vi "stage_move_axis_absolute.vi"(3 "error in":errorcluster, 4 "Ziel xyz IN [mm]":dbl[](array[numeric]), 5 "Achse":i32) -> (0 "error out":errorcluster, 1 "Fertig?":bool, 2 "Ziel xyz OUT [mm]":dbl[](array[numeric]))   [LabVIEW 2009]
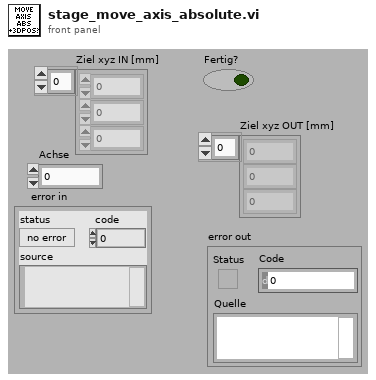
[diagram p1: front panel]
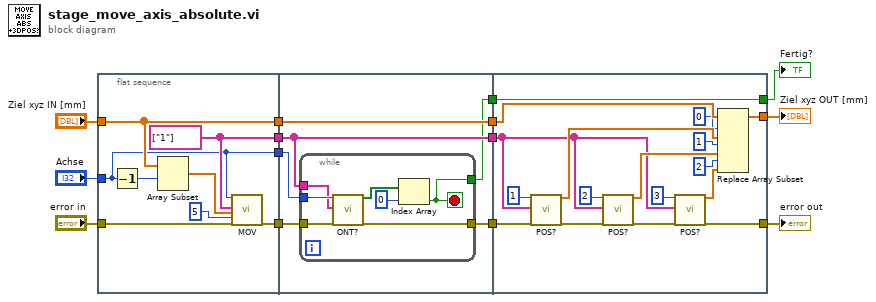
[diagram p0: block diagram]
diagram:
  n1 = flat-sequence {
    tunnel: [w16] -> w14
    tunnel: [w22] -> w13
    tunnel: "Achse" -> [w16]
    tunnel: [w20] -> w12
    tunnel: [w18] -> w7
    tunnel: "Ziel xyz IN [mm]" -> [w18]
    tunnel: "error in" -> [w15]
    tunnel: w14 -> [w28]
    tunnel: w13 -> [w27]
    tunnel: [w26] -> w11
    tunnel: w12 -> [w25]
    tunnel: [w25] -> w10
    tunnel: w7 -> [w24]
    tunnel: [w24] -> w6
    tunnel: [w23] -> w2
    tunnel: w11 -> [w52]
    tunnel: w10 -> [w37]
    tunnel: w6 -> [w49]
    tunnel: [w50] -> w9
    tunnel: [w46] -> w3
    tunnel: w2 -> [w36]
    tunnel: [w36] -> w1
    frame #0 {
      w20 = string[] ["1"] ("Axes to move")
      n2 = Decrement(x=w16) -> (x-1=w17:i32)
      n3 = Array Subset(array=w18, index=w17) -> (w19:dbl[])  [unwired: 1 in]
      n4 = call "MOV.vi"("System no."=w16, "Axes to move"=w20, "Position values"=w19, "No.of digits"=i16 5, "error in"=w15) -> ("error out"=w22:errorcluster)  [unwired: 14 in]
    }
    frame #1 {
      n5 = while {
        tunnel: w28 -> [w35]
        tunnel: w27 -> [w34]
        tunnel: [w33] -> w26
        tunnel: w25 -> [w32]
        tunnel: [w29] -> w23
        stop <- w29 stop-if-true
        n6 = call "ONT?.vi"("System no."=w35, "Axes to query"=w32, "error in"=w34) -> ("Axis on target?"=w30:bool[], "error out"=w33:errorcluster)  [unwired: 15 in]
        n7 = Index Array(array=w30, index=0 ("Index")) -> (element=w29:bool)
      }
    }
    frame #2 {
      n8 = call "POS?.vi"("System no."=1, "Axes to query"=w37, "error in"=w52) -> ("Position"=w51:dbl[], "error out"=w48:errorcluster)  [unwired: 15 in]
      n9 = call "POS?.vi"("System no."=2, "Axes to query"=w37, "error in"=w48) -> ("Position"=w39:dbl[], "error out"=w47:errorcluster)  [unwired: 15 in]
      n10 = call "POS?.vi"("System no."=3, "Axes to query"=w37, "error in"=w47) -> ("Position"=w38:dbl[], "error out"=w46:errorcluster)  [unwired: 15 in]
      n11 = Replace Array Subset(array=w49, new element #1=w51, index #1=0 ("Index"), new element #2=w39, index #2=1 ("Index"), new element #3=w38, index #3=2 ("Index")) -> (w50:dbl[])
    }
  }
  "Ziel xyz OUT [mm]" <- w9
  "error out" <- w3
  "Fertig?" <- w1
